vi "Measurement Data Convert.vi"   [LabVIEW 2016, in "Yokogawa WT300 Series.lvlib"]
doc: "Transforms measurement datas into numeric values."
uses:
  Yokogawa WT300 Series.lvlib
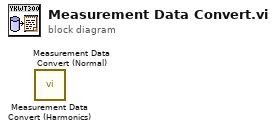
[diagram p0: block diagram]
diagram:
  n1 = call "Measurement Data Convert (Harmonics).vi"() -> ()  [unwired: 8 in, 4 out]
  n2 = call "Measurement Data Convert (Normal).vi"() -> ()  [unwired: 8 in, 4 out]
